vi "Task from tool.vi"(10 "Tool":dbl, 11 "Assignment - Task":string) -> (2 "Task to String":string, 3 "Assignment":string)   [LabVIEW 2022 SP3]
doc: "Assigning robot task, given the previesly selected tool."
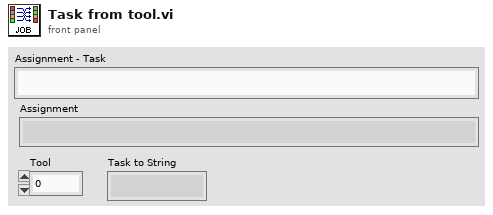
[diagram p1: front panel]
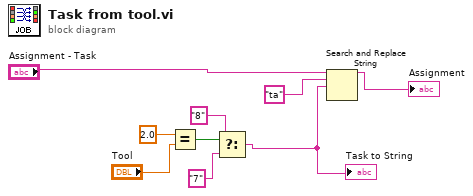
[diagram p0: block diagram]
diagram:
  n1 = Equal?(x=2.0, y="Tool") -> (x = y?=w8:bool)
  n2 = Select(t="8", s=w8, f="7") -> (s? t:f=w3:string)
  "Task to String" <- w3
  n3 = Search and Replace String(input string="Assignment - Task", search string="ta", replace string=w3) -> (result string=→"Assignment":string)  [unwired: 5 in, 3 out]
